vi "Latihan 11 (Enum Case).vi"() -> ()   [LabVIEW 2021]
panel:
  in  "Opsi":enum16{"Customer", "Personal", "Admin"}(ring)
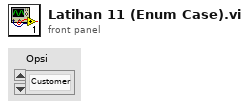
[diagram p1: front panel]
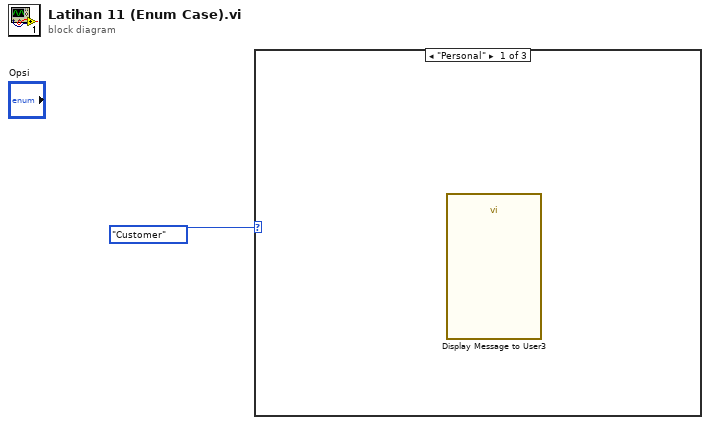
[diagram p0: block diagram]
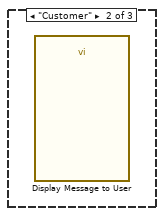
[diagram p2: hidden frame]
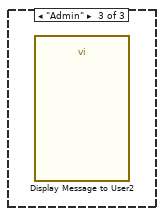
[diagram p3: hidden frame]
diagram:
  n1 = case shown="\"Personal\"" enum16{"Customer", "Personal", "Admin"}."Customer" {
    frame "Personal" {
      n2 = call "Display Message to User3"() -> ()  [unwired: 10 in, 2 out]
    }
    frame "Customer" {
      n3 = call "Display Message to User"() -> ()  [unwired: 10 in, 2 out]
    }
    frame "Admin" {
      n4 = call "Display Message to User2"() -> ()  [unwired: 10 in, 2 out]
    }
  }
